vi "SIGLENT_SPD3303X-E_front_panel.vi"(0 "VISA resource name":refnum<visa-resource-name>, 1 "Knob":dbl(knob) scale=0.0..32.0 scale format="%#.2g", 2 "Volt / Curr":bool, 3 "CH1 / CH2":bool) -> (14 "V CH1":dbl, 15 "I CH1":dbl, 16 "V CH2":dbl, 17 "I CH2":dbl, 19 "error out":errorcluster)   [LabVIEW 2020]
doc: "The application was created for educational purposes, based on the SIGLENT SPD3303X-E power supply.\nTested on the SIGLENT SPD3303X-E power supply.\n\nMade by Piotr Królak"
uses:
  controls/SCPI_enum.ctl
  <vilib>/Utility/file.llb/Write Delimited Spreadsheet (DBL).vi
panel:
  in  "Tab Control":enum32{"CH1", "CH2", "SETTINGS"}(tab)
  in  "ON/OFF CH1":bool
  out "MEASure:VOLTage? CH1 Chart":dbl(graph)
  out "CH1 STATE":bool
  out "V Target CH1":dbl format="%#.2g"
  out "I Target CH1":dbl format="%#.2g"
  in  "ON/OFF CH2":bool
  out "MEASure:VOLTage? CH2 Chart 2":dbl(graph)
  out "CH2 STATE":bool
  out "V Target CH2":dbl format="%#.2g"
  out "I Target CH2":dbl format="%#.2g"
  in  "SCPI":bool
  in  "ZAPISZ":bool
  in  "stop":bool
  in  "POWER":bool
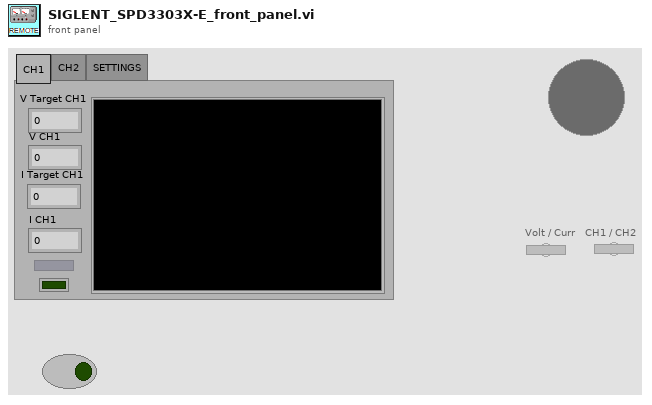
[diagram p1: front panel]
types:
  T1 = typedef "SCPI_enum.ctl" = u16
  T2 = enum8{"Enabled", "Disabled", "Disabled and Grayed Out"}
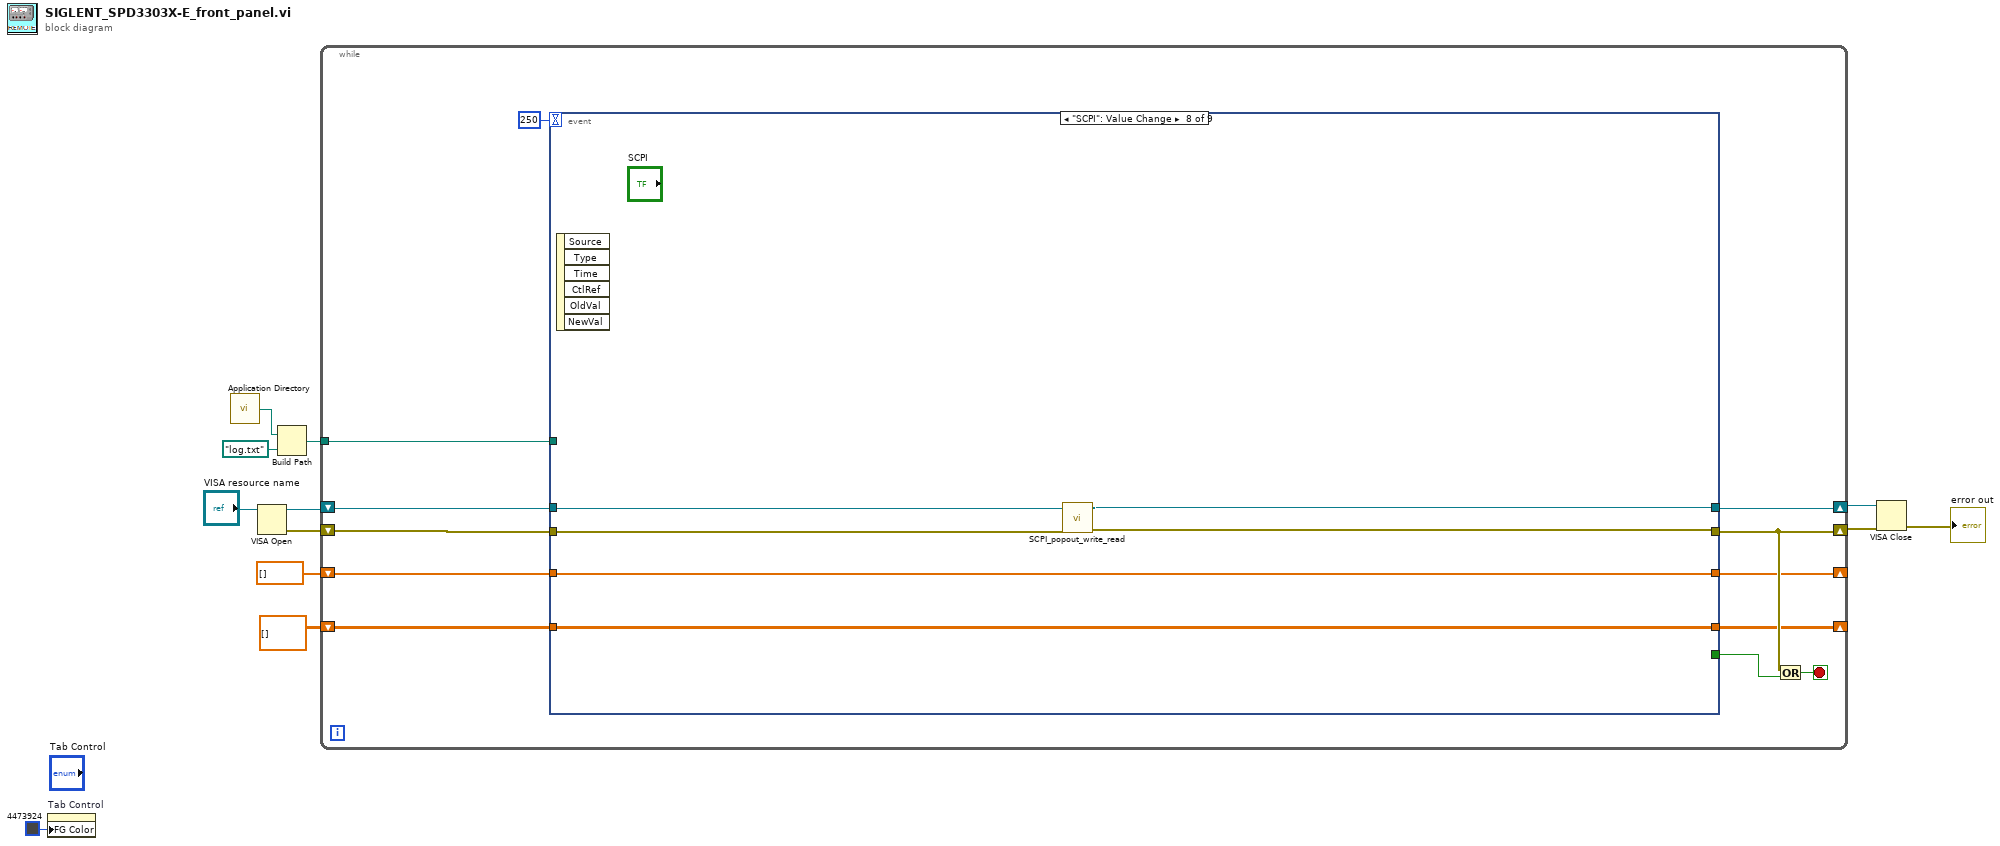
[diagram p0: block diagram]
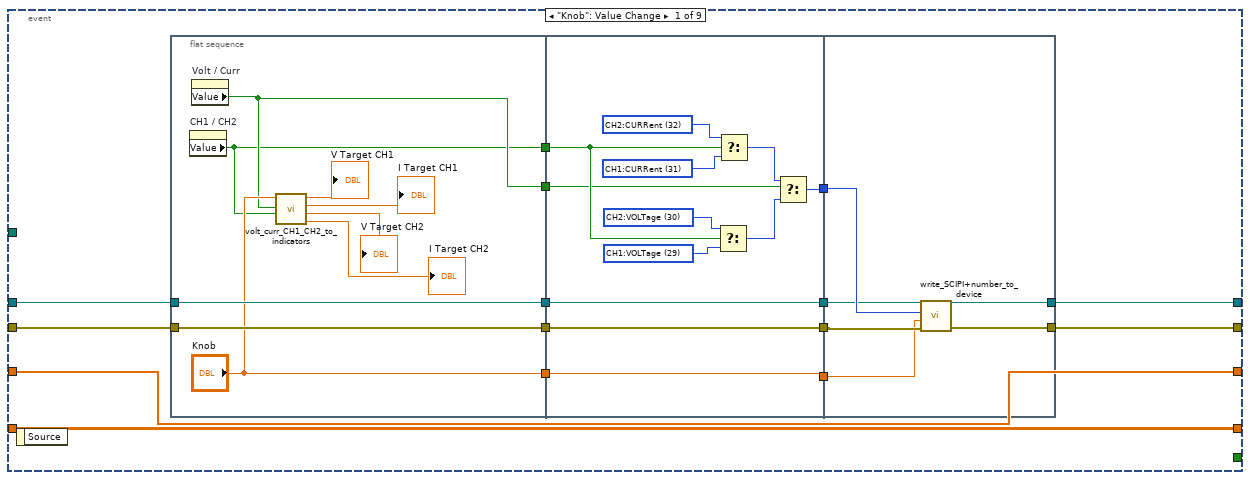
[diagram p2: hidden frame]
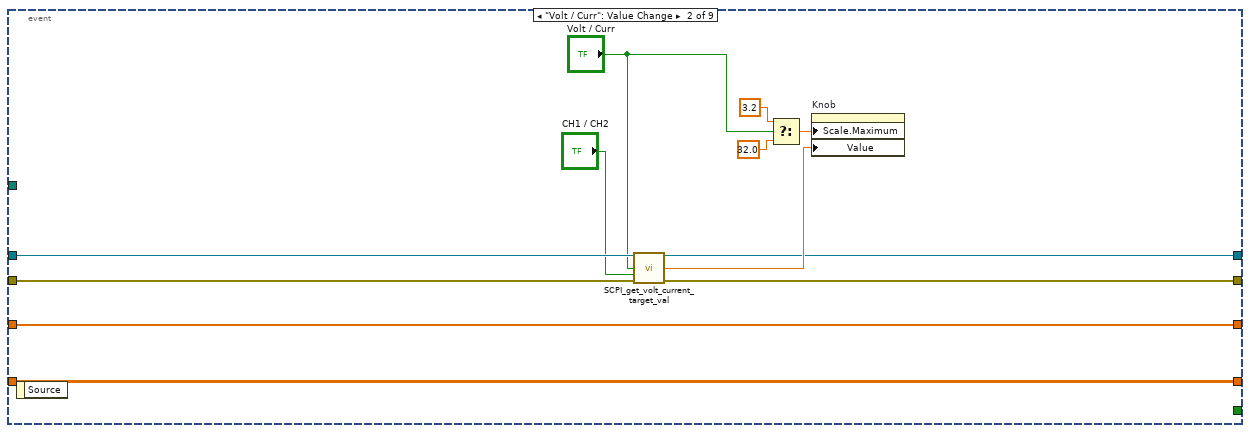
[diagram p3: hidden frame]
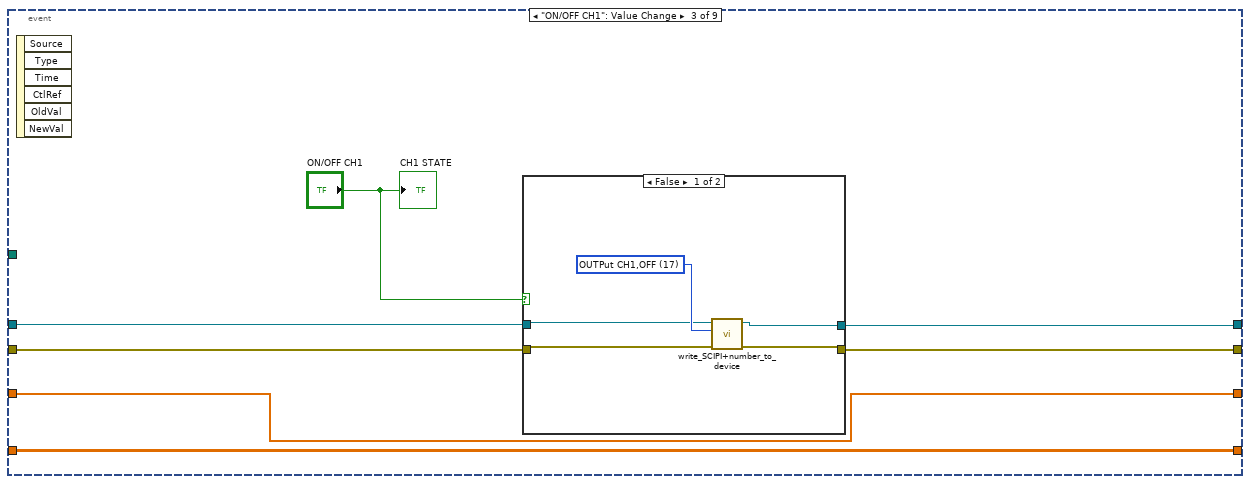
[diagram p4: hidden frame]
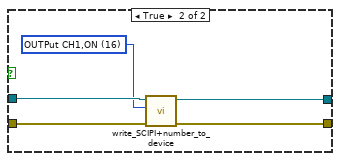
[diagram p5: hidden frame]
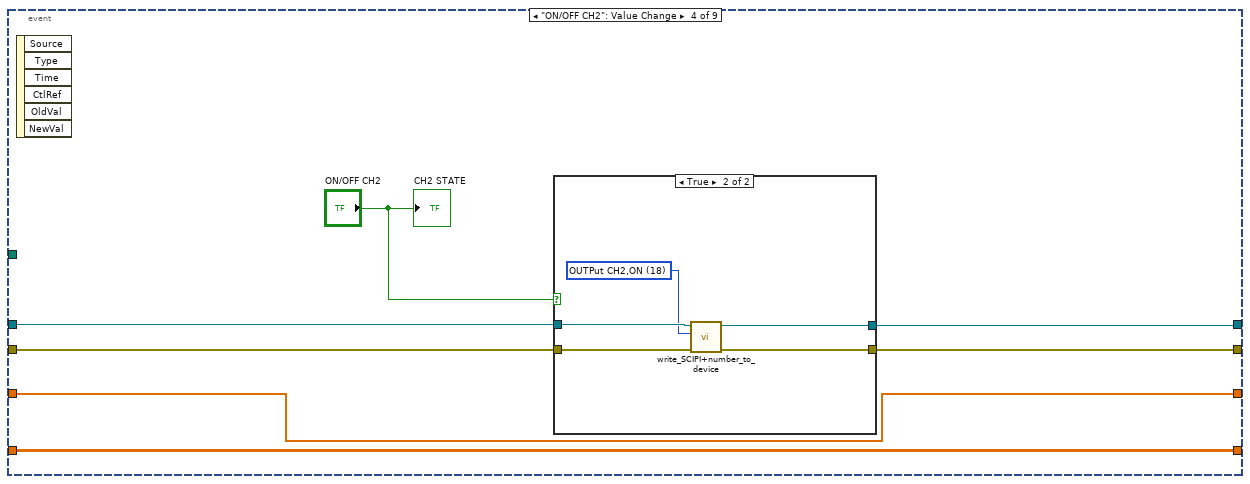
[diagram p6: hidden frame]
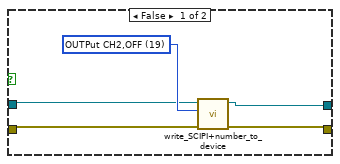
[diagram p7: hidden frame]
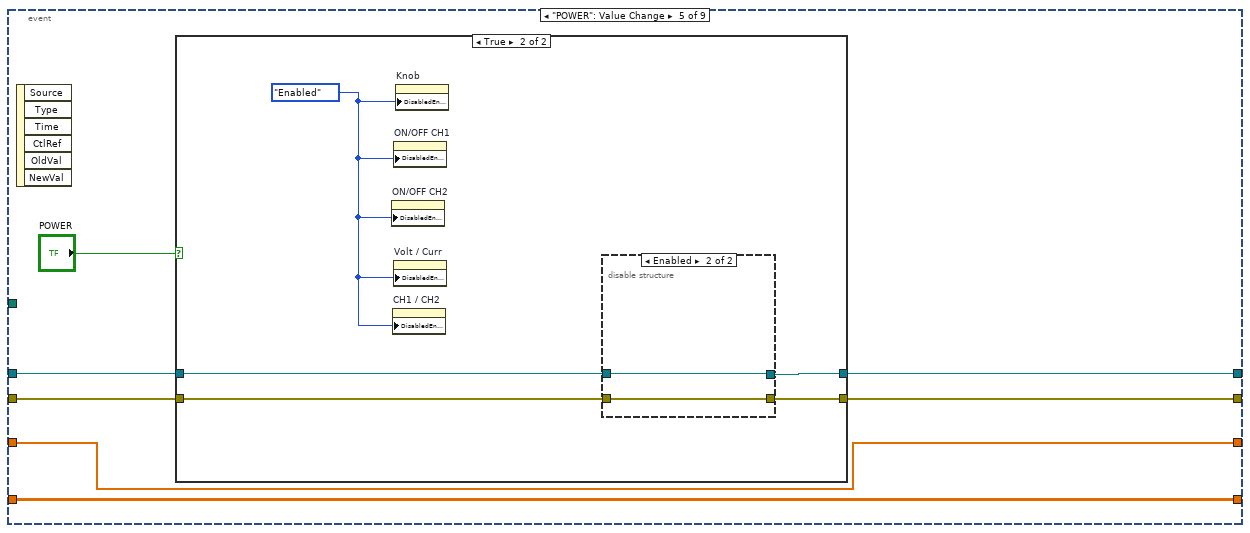
[diagram p8: hidden frame]
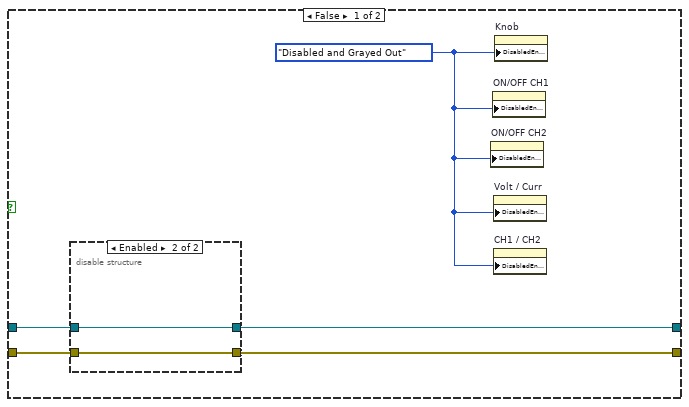
[diagram p9: hidden frame]
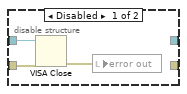
[diagram p10: hidden frame]
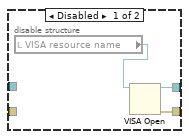
[diagram p11: hidden frame]
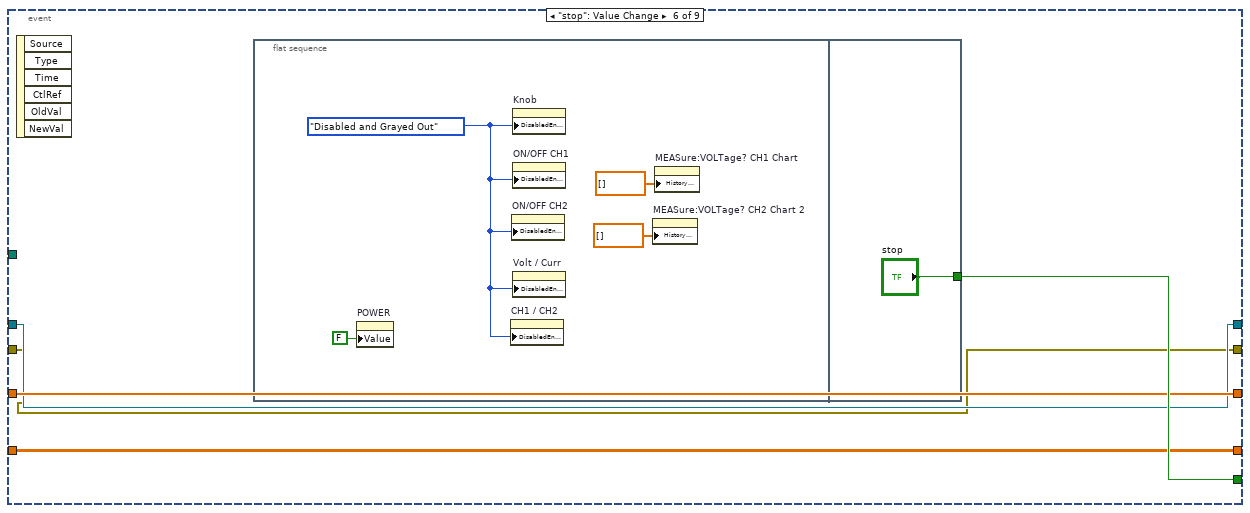
[diagram p12: hidden frame]
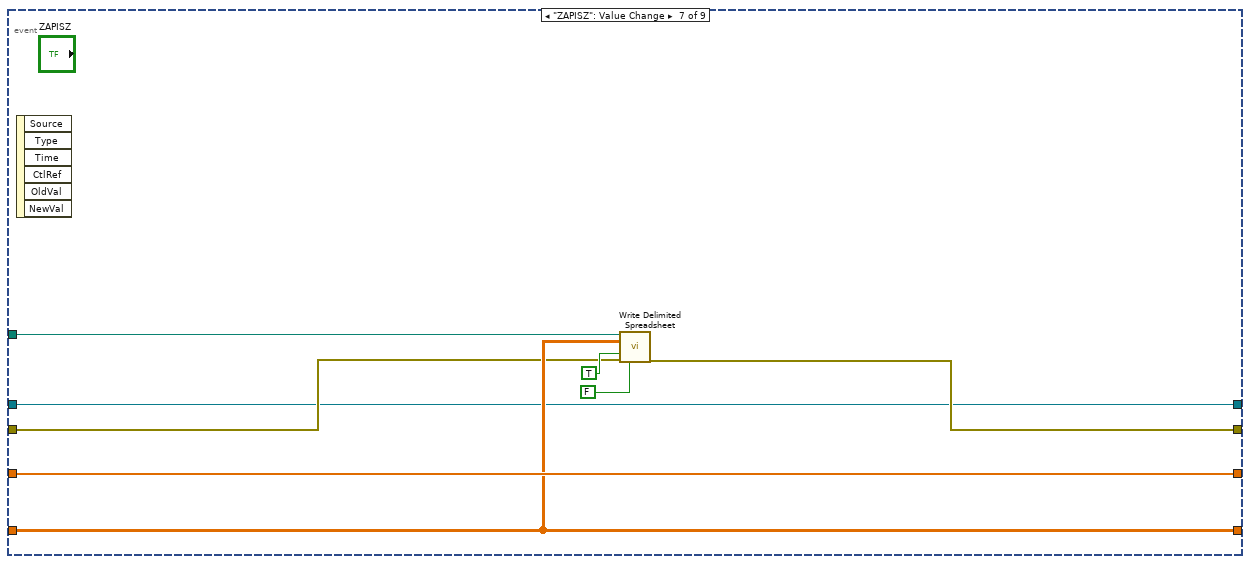
[diagram p13: hidden frame]
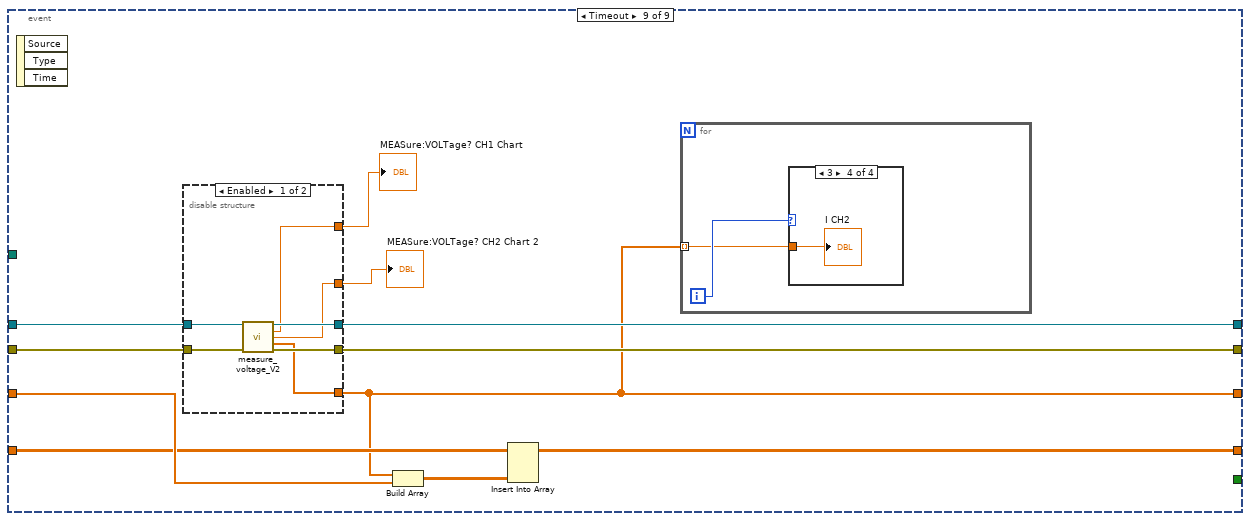
[diagram p14: hidden frame]
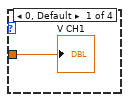
[diagram p15: hidden frame]
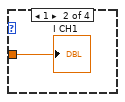
[diagram p16: hidden frame]
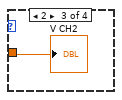
[diagram p17: hidden frame]
diagram:
  n1 = property on="Tab Control" class="TabCtl (strict)"("FG Color"=u32 4473924 ("Colors:FG Color")) -> ()  [unwired: 2 in, 2 out]
  n2 = call <vilib>:"Application Directory.vi"() -> ("Application Directory"=w1:path)
  n3 = VISA Open(VISA resource name="VISA resource name") -> (VISA resource name=w11:refnum<visa-resource-name>, error out=w10:errorcluster)  [unwired: 4 in]
  n4 = Build Path(base path=w1, name or relative path=path "log.txt") -> (appended path=w2:path)
  n5 = while {
    shift-right: [w21] -> w7
    shift-left: w10 -> [w20]
    shift-right: [w22] -> w8
    shift-left: w11 -> [w23]
    shift-right: [w18] -> _
    shift-left: dbl[] [] ("output Array") -> [w16]
    shift-right: [w14] -> _
    shift-left: dbl[][] [] ("appended array") -> [w15]
    tunnel: w2 -> [w13]
    stop <- w24 stop-if-true
    n6 = event shown="[7] \"SCPI\": Value Change" {
      selector: _ -> [_ _ _ _ _ _ _ _ _]
      dyn-events: _ -> [_ _ _ _ _ _ _ _ _]
      timeout: 250 -> [_ _ _ _ _ _ _ _ _]
      tunnel: [_ _ _ _ _ w144 _ _ _] -> w17
      tunnel: w23 -> [w36 w78 w82 w100 w118 w141 w150 w161 w174]
      tunnel: [w39 w72 w85 w99 w116 w141 w150 w159 w172] -> w22
      tunnel: w20 -> [w37 w77 w81 w101 w117 w140 w151 w160 w173]
      tunnel: [w38 w71 w84 w98 w115 w140 w152 w158 w171] -> w21
      tunnel: [w32 w68 w80 w97 w114 w143 w157 w163 w164] -> w18
      tunnel: w16 -> [w32 w68 w80 w97 w114 w143 w157 w163 w170]
      tunnel: [w31 w67 w79 w96 w113 w142 w156 w162 w165] -> w14
      tunnel: w15 -> [w31 w67 w79 w96 w113 w142 w156 w162 w167]
      tunnel: w13 -> [_ _ _ _ _ _ w155 _ _]
      event "Knob": Value Change {
        n7 = event-data() -> ()  [unwired: 1 in, 1 out]
        n8 = flat-sequence {
          tunnel: w36 -> [w47]
          tunnel: w37 -> [w48]
          tunnel: [w48] -> w29
          tunnel: [w47] -> w28
          tunnel: ["Knob"] -> w27
          tunnel: [w44] -> w26
          tunnel: [w45] -> w25
          tunnel: [w54] -> w35
          tunnel: [w53] -> w34
          tunnel: [w52] -> w33
          tunnel: [w51] -> w30
          tunnel: w29 -> [w54]
          tunnel: w28 -> [w52]
          tunnel: w27 -> [w51]
          tunnel: w26 -> [w50]
          tunnel: w25 -> [w49]
          tunnel: [w63] -> w38
          tunnel: [w62] -> w39
          tunnel: w35 -> [w66]
          tunnel: w34 -> [w65]
          tunnel: w33 -> [w64]
          tunnel: w30 -> [w61]
          frame #0 {
            n9 = property on="CH1 / CH2" class="Bool (strict)"() -> ("Value"=w44:bool)  [unwired: 2 in, 2 out]
            n10 = property on="Volt / Curr" class="Bool (strict)"() -> ("Value"=w45:bool)  [unwired: 2 in, 2 out]
            n11 = call "volt_curr_CH1_CH2_to_indicators.vi"("CH1 / CH2"=w44, "Volt / Curr"=w45, "Knob"="Knob") -> ("Current Target CH2"=→"I Target CH2":dbl, "Voltage  Target CH2"=→"V Target CH2":dbl, "Curent Target CH1"=→"I Target CH1":dbl, "Voltage Target CH1"=→"V Target CH1":dbl)  [unwired: 5 in]
          }
          frame #1 {
            w58 = T1 31 items=["*IDN?", "*SAV 1", "*RCL 1", "INSTTrument CH1", "INSTTrument CH2", "INSTrument?", "MEASure:CURRent? CH1", "MEASure:CURRent? CH2", "MEASure:VOLTage? CH1", "MEASure:VOLTage? CH2", "MEASure:POWEr? CH1", "MEASure:POWEr? CH2", "CH1:CURRent?", "CH2:CURRent?", "CH1:VOLTage? ", "CH2:VOLTage? ", "OUTPut CH1,ON", "OUTPut CH1,OFF", "OUTPut CH2,ON", "OUTPut CH2,OFF", "OUTPut CH3,ON", "OUTPut CH3,OFF", "OUTPut:TRACK 0", "OUTPut:TRACK 1", "OUTPut:TRACK 2", "OUTPut:WAVE CH1,ON", "OUTPut:WAVE CH1,OFF", "OUTPut:WAVE CH2,ON", "OUTPut:WAVE CH2,OFF", "CH1:VOLTage", "CH2:VOLTage", "CH1:CURRent", "CH2:CURRent"] ("SCPI")
            w59 = T1 32 items=["*IDN?", "*SAV 1", "*RCL 1", "INSTTrument CH1", "INSTTrument CH2", "INSTrument?", "MEASure:CURRent? CH1", "MEASure:CURRent? CH2", "MEASure:VOLTage? CH1", "MEASure:VOLTage? CH2", "MEASure:POWEr? CH1", "MEASure:POWEr? CH2", "CH1:CURRent?", "CH2:CURRent?", "CH1:VOLTage? ", "CH2:VOLTage? ", "OUTPut CH1,ON", "OUTPut CH1,OFF", "OUTPut CH2,ON", "OUTPut CH2,OFF", "OUTPut CH3,ON", "OUTPut CH3,OFF", "OUTPut:TRACK 0", "OUTPut:TRACK 1", "OUTPut:TRACK 2", "OUTPut:WAVE CH1,ON", "OUTPut:WAVE CH1,OFF", "OUTPut:WAVE CH2,ON", "OUTPut:WAVE CH2,OFF", "CH1:VOLTage", "CH2:VOLTage", "CH1:CURRent", "CH2:CURRent"] ("SCPI")
            w57 = T1 29 items=["*IDN?", "*SAV 1", "*RCL 1", "INSTTrument CH1", "INSTTrument CH2", "INSTrument?", "MEASure:CURRent? CH1", "MEASure:CURRent? CH2", "MEASure:VOLTage? CH1", "MEASure:VOLTage? CH2", "MEASure:POWEr? CH1", "MEASure:POWEr? CH2", "CH1:CURRent?", "CH2:CURRent?", "CH1:VOLTage? ", "CH2:VOLTage? ", "OUTPut CH1,ON", "OUTPut CH1,OFF", "OUTPut CH2,ON", "OUTPut CH2,OFF", "OUTPut CH3,ON", "OUTPut CH3,OFF", "OUTPut:TRACK 0", "OUTPut:TRACK 1", "OUTPut:TRACK 2", "OUTPut:WAVE CH1,ON", "OUTPut:WAVE CH1,OFF", "OUTPut:WAVE CH2,ON", "OUTPut:WAVE CH2,OFF", "CH1:VOLTage", "CH2:VOLTage", "CH1:CURRent", "CH2:CURRent"] ("SCPI")
            w60 = T1 30 items=["*IDN?", "*SAV 1", "*RCL 1", "INSTTrument CH1", "INSTTrument CH2", "INSTrument?", "MEASure:CURRent? CH1", "MEASure:CURRent? CH2", "MEASure:VOLTage? CH1", "MEASure:VOLTage? CH2", "MEASure:POWEr? CH1", "MEASure:POWEr? CH2", "CH1:CURRent?", "CH2:CURRent?", "CH1:VOLTage? ", "CH2:VOLTage? ", "OUTPut CH1,ON", "OUTPut CH1,OFF", "OUTPut CH2,ON", "OUTPut CH2,OFF", "OUTPut CH3,ON", "OUTPut CH3,OFF", "OUTPut:TRACK 0", "OUTPut:TRACK 1", "OUTPut:TRACK 2", "OUTPut:WAVE CH1,ON", "OUTPut:WAVE CH1,OFF", "OUTPut:WAVE CH2,ON", "OUTPut:WAVE CH2,OFF", "CH1:VOLTage", "CH2:VOLTage", "CH1:CURRent", "CH2:CURRent"] ("SCPI")
            n12 = Select(t=w60, s=w50, f=w57) -> (s? t:f=w56:T1)
            n13 = Select(t=w59, s=w50, f=w58) -> (s? t:f=w55:T1)
            n14 = Select(t=w55, s=w49, f=w56) -> (s? t:f=w53:T1)
          }
          frame #2 {
            n15 = call "write_SCIPI+number_to_device.vi"("error in (no error)"=w66, "Numeric"=w61, "SCIPI"=w65, "VISA"=w64) -> ("error out"=w63:errorcluster, "VISA resource name out"=w62:refnum<visa-resource-name>)  [unwired: 6 in]
          }
        }
      }
      event "Volt / Curr": Value Change {
        n16 = event-data() -> ()  [unwired: 1 in, 1 out]
        n17 = call "SCPI_get_volt_current_target_val.vi"("VISA"=w78, "Volt / Curr"="Volt / Curr", "CH1/CH2"="CH1 / CH2", "error in (no error)"=w77) -> ("VISA resource name out"=w72:refnum<visa-resource-name>, "numeric value"=w73:dbl, "error out"=w71:errorcluster)  [unwired: 9 in]
        n18 = Select(t=3.2 ("f"), s="Volt / Curr", f=32.0 ("t")) -> (s? t:f=w76:dbl)
        n19 = property on="Knob" class="Knob (strict)"("Scale.Maximum"=w76, "Value"=w73) -> ()  [unwired: 2 in, 2 out]
      }
      event "ON/OFF CH1": Value Change {
        n20 = event-data() -> ()  [unwired: 1 in, 6 out]
        n21 = case shown="False" "ON/OFF CH1" {
          tunnel: w81 -> [w86 w95]
          tunnel: w82 -> [w87 w94]
          tunnel: [w89 w93] -> w85
          tunnel: [w88 w92] -> w84
          frame False {
            w90 = T1 17 items=["*IDN?", "*SAV 1", "*RCL 1", "INSTTrument CH1", "INSTTrument CH2", "INSTrument?", "MEASure:CURRent? CH1", "MEASure:CURRent? CH2", "MEASure:VOLTage? CH1", "MEASure:VOLTage? CH2", "MEASure:POWEr? CH1", "MEASure:POWEr? CH2", "CH1:CURRent?", "CH2:CURRent?", "CH1:VOLTage? ", "CH2:VOLTage? ", "OUTPut CH1,ON", "OUTPut CH1,OFF", "OUTPut CH2,ON", "OUTPut CH2,OFF", "OUTPut CH3,ON", "OUTPut CH3,OFF", "OUTPut:TRACK 0", "OUTPut:TRACK 1", "OUTPut:TRACK 2", "OUTPut:WAVE CH1,ON", "OUTPut:WAVE CH1,OFF", "OUTPut:WAVE CH2,ON", "OUTPut:WAVE CH2,OFF", "CH1:VOLTage", "CH2:VOLTage", "CH1:CURRent", "CH2:CURRent"] ("SCIPI")
            n22 = call "write_SCIPI+number_to_device.vi"("error in (no error)"=w86, "SCIPI"=w90, "VISA"=w87) -> ("error out"=w88:errorcluster, "VISA resource name out"=w89:refnum<visa-resource-name>)  [unwired: 7 in]
          }
          frame True {
            w91 = T1 16 items=["*IDN?", "*SAV 1", "*RCL 1", "INSTTrument CH1", "INSTTrument CH2", "INSTrument?", "MEASure:CURRent? CH1", "MEASure:CURRent? CH2", "MEASure:VOLTage? CH1", "MEASure:VOLTage? CH2", "MEASure:POWEr? CH1", "MEASure:POWEr? CH2", "CH1:CURRent?", "CH2:CURRent?", "CH1:VOLTage? ", "CH2:VOLTage? ", "OUTPut CH1,ON", "OUTPut CH1,OFF", "OUTPut CH2,ON", "OUTPut CH2,OFF", "OUTPut CH3,ON", "OUTPut CH3,OFF", "OUTPut:TRACK 0", "OUTPut:TRACK 1", "OUTPut:TRACK 2", "OUTPut:WAVE CH1,ON", "OUTPut:WAVE CH1,OFF", "OUTPut:WAVE CH2,ON", "OUTPut:WAVE CH2,OFF", "CH1:VOLTage", "CH2:VOLTage", "CH1:CURRent", "CH2:CURRent"] ("SCIPI")
            n23 = call "write_SCIPI+number_to_device.vi"("error in (no error)"=w95, "SCIPI"=w91, "VISA"=w94) -> ("error out"=w92:errorcluster, "VISA resource name out"=w93:refnum<visa-resource-name>)  [unwired: 7 in]
          }
        }
        "CH1 STATE" <- "ON/OFF CH1"
      }
      event "ON/OFF CH2": Value Change {
        n24 = event-data() -> ()  [unwired: 1 in, 6 out]
        n25 = case shown="True" "ON/OFF CH2" {
          tunnel: w101 -> [w103 w112]
          tunnel: w100 -> [w104 w111]
          tunnel: [w106 w110] -> w99
          tunnel: [w105 w109] -> w98
          frame False {
            w107 = T1 19 items=["*IDN?", "*SAV 1", "*RCL 1", "INSTTrument CH1", "INSTTrument CH2", "INSTrument?", "MEASure:CURRent? CH1", "MEASure:CURRent? CH2", "MEASure:VOLTage? CH1", "MEASure:VOLTage? CH2", "MEASure:POWEr? CH1", "MEASure:POWEr? CH2", "CH1:CURRent?", "CH2:CURRent?", "CH1:VOLTage? ", "CH2:VOLTage? ", "OUTPut CH1,ON", "OUTPut CH1,OFF", "OUTPut CH2,ON", "OUTPut CH2,OFF", "OUTPut CH3,ON", "OUTPut CH3,OFF", "OUTPut:TRACK 0", "OUTPut:TRACK 1", "OUTPut:TRACK 2", "OUTPut:WAVE CH1,ON", "OUTPut:WAVE CH1,OFF", "OUTPut:WAVE CH2,ON", "OUTPut:WAVE CH2,OFF", "CH1:VOLTage", "CH2:VOLTage", "CH1:CURRent", "CH2:CURRent"] ("SCIPI")
            n26 = call "write_SCIPI+number_to_device.vi"("error in (no error)"=w103, "SCIPI"=w107, "VISA"=w104) -> ("error out"=w105:errorcluster, "VISA resource name out"=w106:refnum<visa-resource-name>)  [unwired: 7 in]
          }
          frame True {
            w108 = T1 18 items=["*IDN?", "*SAV 1", "*RCL 1", "INSTTrument CH1", "INSTTrument CH2", "INSTrument?", "MEASure:CURRent? CH1", "MEASure:CURRent? CH2", "MEASure:VOLTage? CH1", "MEASure:VOLTage? CH2", "MEASure:POWEr? CH1", "MEASure:POWEr? CH2", "CH1:CURRent?", "CH2:CURRent?", "CH1:VOLTage? ", "CH2:VOLTage? ", "OUTPut CH1,ON", "OUTPut CH1,OFF", "OUTPut CH2,ON", "OUTPut CH2,OFF", "OUTPut CH3,ON", "OUTPut CH3,OFF", "OUTPut:TRACK 0", "OUTPut:TRACK 1", "OUTPut:TRACK 2", "OUTPut:WAVE CH1,ON", "OUTPut:WAVE CH1,OFF", "OUTPut:WAVE CH2,ON", "OUTPut:WAVE CH2,OFF", "CH1:VOLTage", "CH2:VOLTage", "CH1:CURRent", "CH2:CURRent"] ("SCIPI")
            n27 = call "write_SCIPI+number_to_device.vi"("error in (no error)"=w112, "SCIPI"=w108, "VISA"=w111) -> ("error out"=w109:errorcluster, "VISA resource name out"=w110:refnum<visa-resource-name>)  [unwired: 7 in]
          }
        }
        "CH2 STATE" <- "ON/OFF CH2"
      }
      event "POWER": Value Change {
        n28 = event-data() -> ()  [unwired: 1 in, 6 out]
        n29 = case shown="True" "POWER" {
          tunnel: w118 -> [w124 w130]
          tunnel: w117 -> [w123 w131]
          tunnel: [w121 w134] -> w116
          tunnel: [w120 w133] -> w115
          frame False {
            w122 = T2."Disabled and Grayed Out" ("Disabled")
            n30 = disable-structure shown="Enabled" {
              disable-tunnel: w124 -> [w127 w129]
              disable-tunnel: w123 -> [w126 w128]
              disable-tunnel: [_ w129] -> w121
              disable-tunnel: [_ w128] -> w120
              frame Disabled {
                n31 = VISA Close(VISA resource name=w127, error in (no error)=w126) -> (error out=w125:errorcluster)
                n32 = local write "error out"(w125) -> ()
              }
              frame Enabled {
              }
            }
            n33 = property on="ON/OFF CH2" class="Bool (strict)"("DisabledEnum"=w122) -> ()  [unwired: 2 in, 2 out]
            n34 = property on="ON/OFF CH1" class="Bool (strict)"("DisabledEnum"=w122) -> ()  [unwired: 2 in, 2 out]
            n35 = property on="Volt / Curr" class="Bool (strict)"("DisabledEnum"=w122) -> ()  [unwired: 2 in, 2 out]
            n36 = property on="CH1 / CH2" class="Bool (strict)"("DisabledEnum"=w122) -> ()  [unwired: 2 in, 2 out]
            n37 = property on="Knob" class="Knob (strict)"("DisabledEnum"=w122) -> ()  [unwired: 2 in, 2 out]
          }
          frame True {
            w132 = T2."Enabled" ("Disabled")
            n38 = property on="ON/OFF CH2" class="Bool (strict)"("DisabledEnum"=w132) -> ()  [unwired: 2 in, 2 out]
            n39 = property on="CH1 / CH2" class="Bool (strict)"("DisabledEnum"=w132) -> ()  [unwired: 2 in, 2 out]
            n40 = property on="ON/OFF CH1" class="Bool (strict)"("DisabledEnum"=w132) -> ()  [unwired: 2 in, 2 out]
            n41 = property on="Volt / Curr" class="Bool (strict)"("DisabledEnum"=w132) -> ()  [unwired: 2 in, 2 out]
            n42 = property on="Knob" class="Knob (strict)"("DisabledEnum"=w132) -> ()  [unwired: 2 in, 2 out]
            n43 = disable-structure shown="Enabled" {
              disable-tunnel: [w137 w138] -> w134
              disable-tunnel: [w136 w139] -> w133
              disable-tunnel: w131 -> [_ w139]
              disable-tunnel: w130 -> [_ w138]
              frame Disabled {
                n44 = local read "VISA resource name"() -> (w135:refnum<visa-resource-name>)
                n45 = VISA Open(VISA resource name=w135) -> (VISA resource name=w137:refnum<visa-resource-name>, error out=w136:errorcluster)  [unwired: 4 in]
              }
              frame Enabled {
              }
            }
          }
        }
      }
      event "stop": Value Change {
        n46 = event-data() -> ()  [unwired: 1 in, 6 out]
        n47 = flat-sequence {
          tunnel: ["stop"] -> w144
          frame #0 {
            w147 = T2."Disabled and Grayed Out" ("Disabled")
            n48 = property on="POWER" class="Bool (strict)"("Value"=FALSE ("POWER")) -> ()  [unwired: 2 in, 2 out]
            n49 = property on="CH1 / CH2" class="Bool (strict)"("DisabledEnum"=w147) -> ()  [unwired: 2 in, 2 out]
            n50 = property on="ON/OFF CH2" class="Bool (strict)"("DisabledEnum"=w147) -> ()  [unwired: 2 in, 2 out]
            n51 = property on="Knob" class="Knob (strict)"("DisabledEnum"=w147) -> ()  [unwired: 2 in, 2 out]
            n52 = property on="ON/OFF CH1" class="Bool (strict)"("DisabledEnum"=w147) -> ()  [unwired: 2 in, 2 out]
            n53 = property on="Volt / Curr" class="Bool (strict)"("DisabledEnum"=w147) -> ()  [unwired: 2 in, 2 out]
            n54 = property on="MEASure:VOLTage? CH2 Chart 2" class="WFChart (strict)"("History Data"=dbl[] []) -> ()  [unwired: 2 in, 2 out]
            n55 = property on="MEASure:VOLTage? CH1 Chart" class="WFChart (strict)"("History Data"=dbl[] []) -> ()  [unwired: 2 in, 2 out]
          }
          frame #1 {
          }
        }
      }
      event "ZAPISZ": Value Change {
        n56 = event-data() -> ()  [unwired: 1 in, 6 out]
        n57 = call-poly <vilib>:"Write Delimited Spreadsheet.vi"("file path (dialog if empty)"=w155, "2D data"=w156, "append to file? (new file:F)"=TRUE, "error in (no error)"=w151, "transpose? (no:F)"=FALSE) -> ("error out"=w152:errorcluster)  [unwired: 9 in, 1 out]
      }
      event "SCPI": Value Change {
        n58 = event-data() -> ()  [unwired: 1 in, 6 out]
        n59 = call "SCPI_popout_write_read.vi"("error in (no error)"=w160, "VISA"=w161) -> ("error out"=w158:errorcluster, "VISA resource name out"=w159:refnum<visa-resource-name>)  [unwired: 8 in]
      }
      event Timeout {
        n60 = event-data() -> ()  [unwired: 1 in, 3 out]
        n61 = disable-structure shown="Enabled" {
          disable-tunnel: w174 -> [w187 w189]
          disable-tunnel: w173 -> [w186 w188]
          disable-tunnel: [w185 w189] -> w172
          disable-tunnel: [w184 w188] -> w171
          disable-tunnel: [w183 _] -> w169
          disable-tunnel: [w182 _] -> w168
          disable-tunnel: [w181 _] -> w164
          frame Enabled {
            n62 = call "measure_voltage_V2.vi"("VISA resource name"=w187, "error in"=w186) -> ("VISA resource name out"=w185:refnum<visa-resource-name>, "MEASure:VOLTage? CH1 Chart"=w183:dbl, "MEASure:VOLTage? CH2 Chart"=w182:dbl, "output Array"=w181:dbl[], "error out"=w184:errorcluster)  [unwired: 9 in]
          }
          frame Disabled {
          }
        }
        "MEASure:VOLTage? CH2 Chart 2" <- w168
        "MEASure:VOLTage? CH1 Chart" <- w169
        n63 = Build Array(w164, w170) -> (w166:dbl[][])
        n64 = Insert Into Array(array=w167, new element=w166) -> (w165:dbl[][])  [unwired: 2 in]
        n65 = for {
          tunnel: w164 -> [w175] mode=indexing
          i -> [w176]
          n66 = case shown="3" w176 {
            tunnel: w175 -> [w177 w178 w179 w180]
            frame 0, Default {
              "V CH1" <- w177
            }
            frame 1 {
              "I CH1" <- w178
            }
            frame 2 {
              "V CH2" <- w179
            }
            frame 3 {
              "I CH2" <- w180
            }
          }
        }
      }
    }
    n67 = Or(x=w21, y=w17) -> (x .or. y?=w24:bool)
  }
  n68 = VISA Close(VISA resource name=w8, error in (no error)=w7) -> (error out=→"error out":errorcluster)
